vi "stepper driver -- IMS -- progress monitor.vi"(8 "talkback user event":refnum<user-event>, 11 "talkto user event":refnum<user-event>) -> ()   [LabVIEW 2018]
uses:
  stepper motor state.ctl
  stepper monitor message.ctl
  talkto async routine actionn.ctl
  stepper motor action.ctl
panel:
  in  "stepper state":T1=enum."stopped"
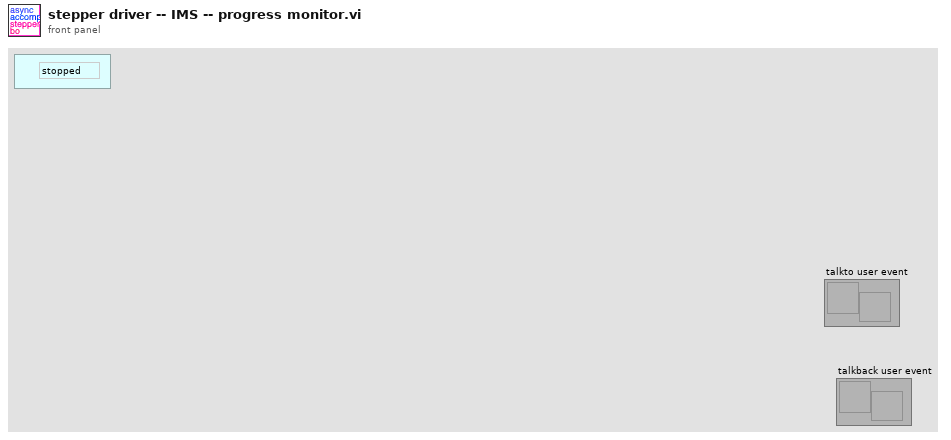
[diagram p1: front panel]
types:
  T1 = typedef "stepper motor state.ctl" = enum16{"moving", "stopped"}
  T2 = typedef "talkto async routine actionn.ctl" = enum16{"stop", "check"}
  T3 = typedef "stepper monitor message.ctl" = cluster{"current position":dbl, "stepper motor state OUT":T1}
  T4 = typedef "stepper motor action.ctl" = enum16{"go", "void", "stop", "check", "init", "sync", "set", "set speed", "--check status", "--check value"}
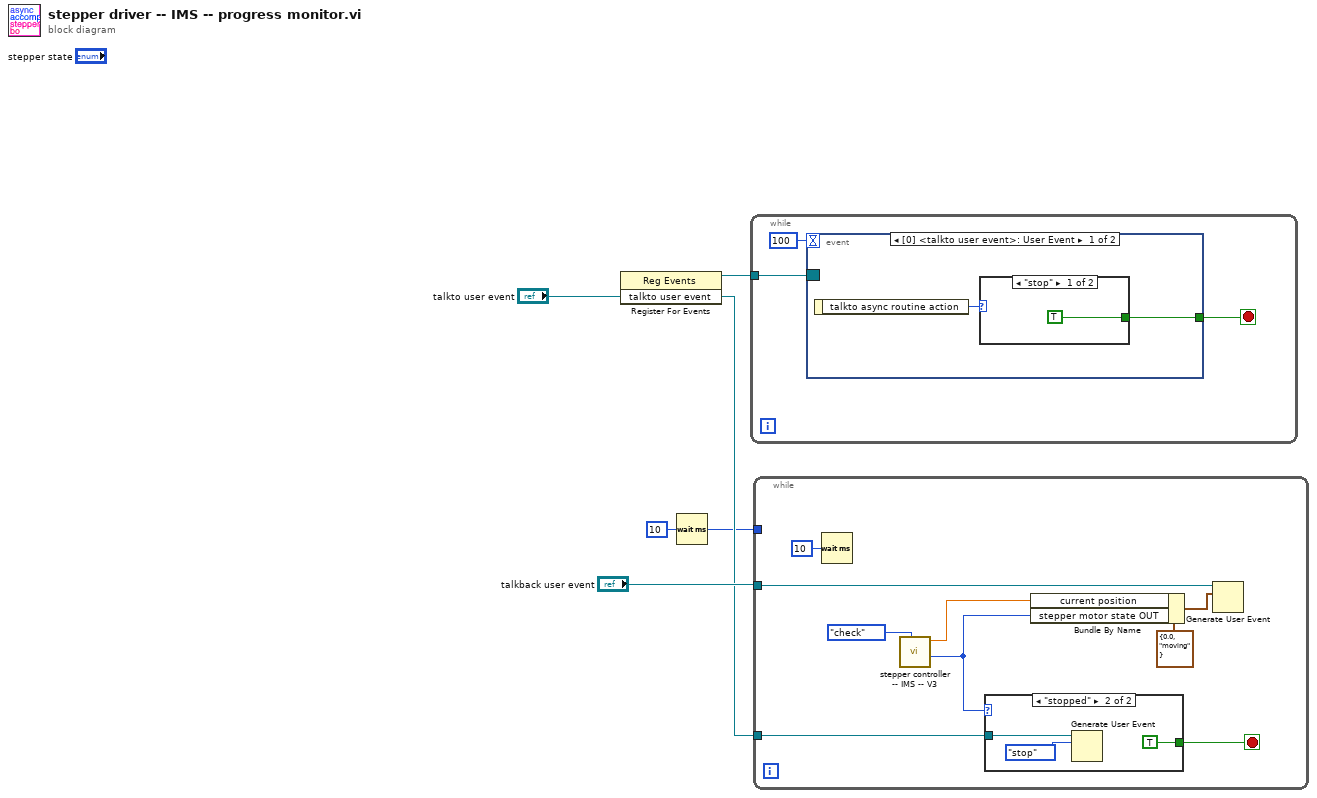
[diagram p0: block diagram]
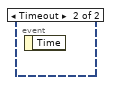
[diagram p3: hidden frame]
diagram:
  n1 = register-events("talkto user event") -> (reference out=w3:refnum<event-registration>)  [unwired: 2 in, 1 out]
  n2 = Wait (ms)(milliseconds to wait=u32 10) -> (millisecond timer value=w1:u32)
  n3 = while {
    tunnel: w3 -> [w8]
    stop <- w6 stop-if-true
    n4 = event shown="[0] <talkto user event>: User Event" {
      selector: w8 -> [_ _]
      dyn-events: _ -> [_ _]
      timeout: 100 -> [_ _]
      tunnel: [w9 _] -> w6
      event User Event {
        n5 = event-data() -> ("talkto async routine action"=w10:T2)  [unwired: 1 in]
        n6 = case shown="\"stop\"" w10 {
          tunnel: [TRUE _] -> w9
          frame "stop" {
          }
          frame "check", Default {
          }
        }
      }
      event Timeout {
        n7 = event-data() -> ()  [unwired: 1 in, 1 out]
      }
    }
  }
  n8 = while {
    tunnel: "talkback user event" -> [w20]
    tunnel: "talkto user event" -> [w17]
    tunnel: w1 -> [_]
    stop <- w16 stop-if-true
    # "This loop is a consumer loop."
    n9 = Wait (ms)(milliseconds to wait=u32 10) -> ()  [unwired: 1 out]
    n10 = call "stepper controller -- IMS -- V3.vi"("stepper driver action"=stepper_motor_action."check") -> ("stepper motor state OUT"=w18:T1, "current position"=w19:dbl)  [unwired: 8 in, 1 out]
    n11 = case shown="\"stopped\"" w18 {
      tunnel: w17 -> [_ w23]
      tunnel: [_ TRUE] -> w16
      frame "moving", Default {
      }
      frame "stopped" {
        n12 = Generate User Event(user event=w23, event data cluster=talkto_async_routine_actionn."stop" ("event data")) -> ()  [unwired: 2 in, 2 out]
      }
    }
    n13 = Bundle By Name(cluster=T3 {"current position"=0.0, "stepper motor state OUT"=enum."moving"} ("stepper monitor message"), "current position"=w19, "stepper motor state OUT"=w18) -> (w13:T3)
    n14 = Generate User Event(user event=w20, event data cluster=w13) -> ()  [unwired: 2 in, 2 out]
  }
